vi "报警信息.vi"(8 "error in (no error)":errorcluster, 11 "data in":T1) -> (0 "error out":errorcluster)   [LabVIEW 2016, in "德润超标留样.lvlib"]
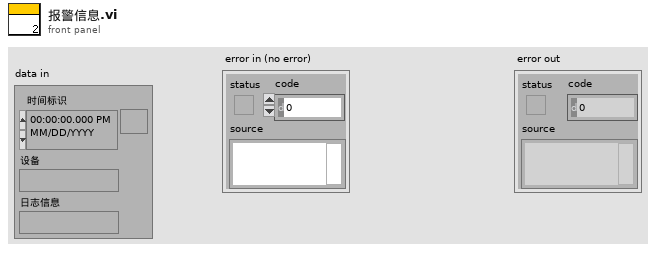
[diagram p1: front panel]
types:
  T1 = cluster{"时间标识":timestamp, "设备":string, "日志信息":string}
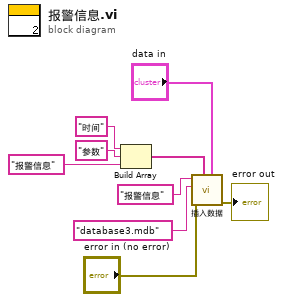
[diagram p0: block diagram]
diagram:
  n1 = Build Array("时间", "参数" ("元素"), "报警信息") -> (w6:string[])
  n2 = call "插入数据.vi"("data"="data in", "columns"=w6, "error in (no error)"="error in (no error)", "database"="database3.mdb", "table"="报警信息") -> ("error out"=→"error out":errorcluster)  [unwired: 6 in]
